vi "wektorowy kalkulator.vi"() -> ()   [LabVIEW 2020]
uses:
  <vilib>/Analysis/NI_AALBase.lvlib
  <vilib>/Analysis/baseanly.llb/Real Dot Product.vi
  <vilib>/Analysis/NI_AALPro.lvlib
panel:
  out "Array 2":dbl[](array[numeric])
  in  "Wektor b":dbl[](array[numeric])
  in  "Wektor a":dbl[](array[numeric])
  in  "Ring":u16(ring) items=["Dodawanie", "Odejmowanie", "Skalarne mnozenie", "Wektorowe mnozenie"]
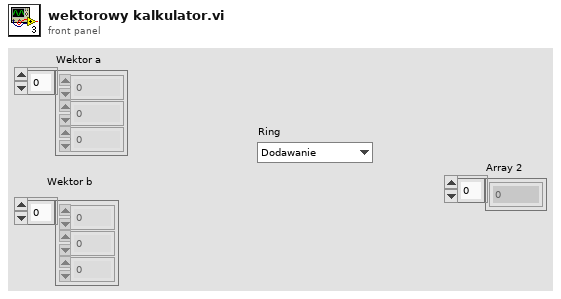
[diagram p1: front panel]
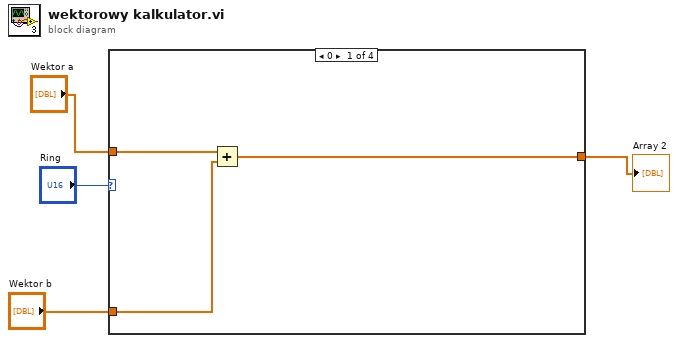
[diagram p0: block diagram]
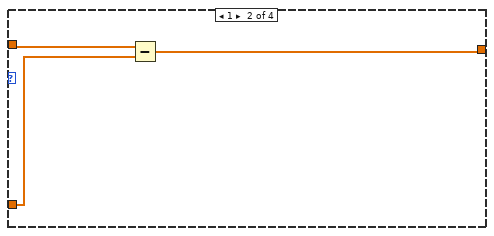
[diagram p2: hidden frame]
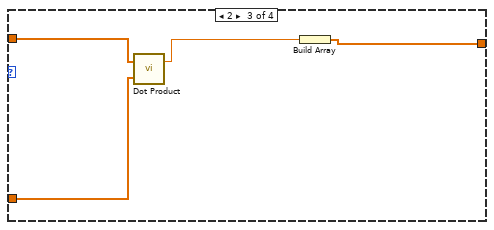
[diagram p3: hidden frame]
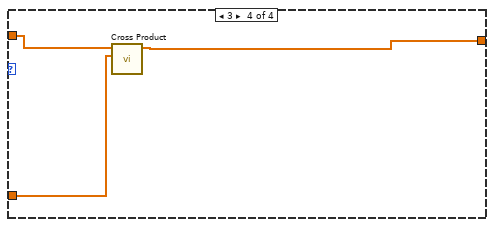
[diagram p4: hidden frame]
diagram:
  n1 = case shown="0" "Ring" {
    tunnel: "Wektor a" -> [w7 w10 w14 w17]
    tunnel: "Wektor b" -> [w6 w9 w13 w16]
    tunnel: [w5 w8 w11 w15] -> w1
    frame 0 {
      n2 = Add(x=w7, y=w6) -> (x+y=w5:dbl[])
    }
    frame 1 {
      n3 = Subtract(x=w10, y=w9) -> (x-y=w8:dbl[])
    }
    frame 2 {
      n4 = call-poly <vilib>:"Dot Product.vi"("Y Vector"=w13, "X Vector"=w14) -> ("X * Y"=w12:dbl)  [unwired: 1 out]
      n5 = Build Array(w12) -> (w11:dbl[])
    }
    frame 3 {
      n6 = call <vilib>:"Cross Product.vi"("B Vector"=w16, "A Vector"=w17) -> ("Cross Product"=w15:dbl[])  [unwired: 8 in, 1 out]
    }
  }
  "Array 2" <- w1
